vi "RM.getAllClientInfo.vi"(8 "error in":errorcluster, 11 "Item Ref in":T2 format="%.0x") -> (0 "error out":errorcluster, 2 "ClientInfo Array":T1[](array[typedef]) {"CD Ref" format="%.0x"}, 3 "Item Ref out":T2 format="%.0x")   [LabVIEW 2016, in "FPGA Resource Manager.lvlib"]
uses:
  <vilib>/NI Veristand/Custom Device API/Custom Device Item Ref.ctl
  RM.clientInfo.ctl
  FPGA Resource Manager.lvlib
  <vilib>/NI Veristand/Custom Device API/Custom Device API.lvlib
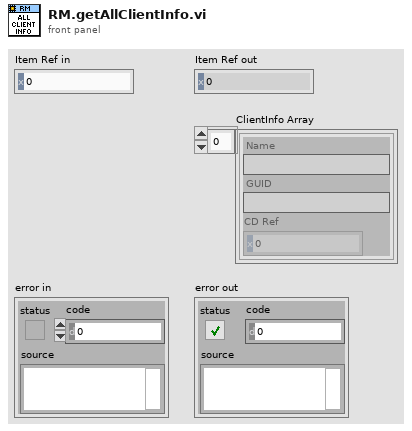
[diagram p1: front panel]
types:
  T1 = typedef "FPGA Resource Manager.lvlib/RM.clientInfo.ctl" = cluster{"Name":string, "GUID":string, "CD Ref":T2}
  T2 = typedef "Custom Device API.lvlib/Custom Device Item Ref.ctl" = u64
  T3 = typedef "Custom Device API.lvlib/Custom Device Item Info.ctl" = cluster{"Name":string, "Is Channel":bool, "GUID":string, "Is Waveform":bool}
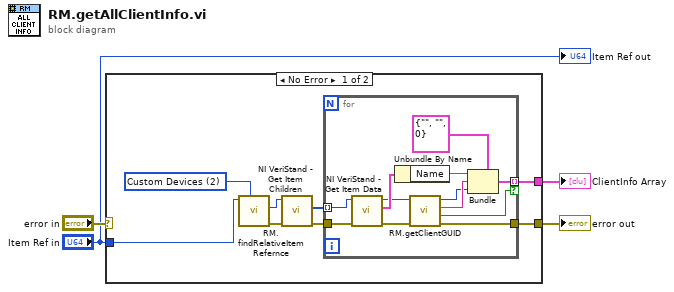
[diagram p0: block diagram]
diagram:
  n1 = case shown="No Error" "error in" {
    selector: "error in" -> [_ w25]
    tunnel: "Item Ref in" -> [w10 _]
    tunnel: [w12 w25] -> w3
    tunnel: [w6 _] -> w1
    frame No Error {
      w11 = u16 2 items=["Targets", "Controller", "Custom Devices", "This CD", "This CD/Group", "This CD/Group/SubGroup"] ("Relative Type")
      n2 = call "RM.findRelativeItemRefernce.vi"("Relative Type"=w11, "Item Ref in"=w10) -> ("error out"=w9:errorcluster, "Relative Item Ref Out"=w8:T2)  [unwired: 5 in, 3 out]
      n3 = call <vilib>:"NI VeriStand - Get Item Children.vi"("error in (no error)"=w9, "Item Ref in"=w8) -> ("error out"=w5:errorcluster, "Child Refs"=w7:T2[])  [unwired: 6 in, 2 out]
      n4 = for {
        tunnel: [w17] -> w12
        tunnel: w7 -> [w24] mode=indexing
        tunnel: [w19] -> w6 mode=indexing if=w13
        tunnel: w5 -> [w22]
        n5 = call <vilib>:"NI VeriStand - Get Item Data.vi"("error in (no error)"=w22, "Item Ref in"=w24) -> ("error out"=w18:errorcluster, "Item Info"=w23:T3, "Item Ref out"=w16:T2)  [unwired: 6 in, 1 out]
        n6 = Unbundle By Name(w23) -> ("Name"=w21:string)
        n7 = call "RM.getClientGUID.vi"("error in (no error)"=w18, "Item Ref in"=w16) -> ("error out"=w17:errorcluster, "Found?"=w13:bool, "ClientGUID"=w15:string, "Item Ref out"=w14:T2)  [unwired: 6 in]
        n8 = Bundle(cluster=T1 {"Name"="", "GUID"="", "CD Ref"=0} ("ClientInfo"), "Name"=w21, "GUID"=w15, "CD Ref"=w14) -> (w19:T1)
      }
    }
    frame Error {
    }
  }
  "error out" <- w3
  "ClientInfo Array" <- w1
  "Item Ref out" <- "Item Ref in"
